vi "Create 3D Sphere.vi"(1 "Radius":sgl, 2 "Color":T1, 3 "Name":string) -> (0 "Scene:New Object":refnum<vi>)   [LabVIEW 2010]
uses:
  <vilib>/picture/3D Picture Control/NI_3D Picture Control.lvlib
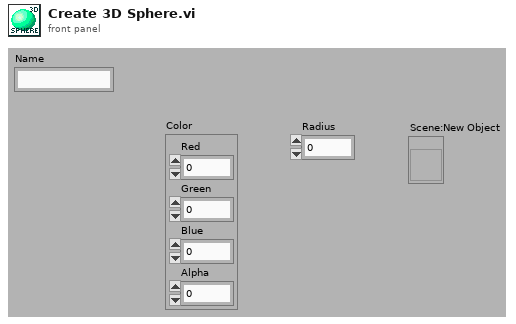
[diagram p1: front panel]
types:
  T1 = cluster{"Red":sgl, "Green":sgl, "Blue":sgl, "Alpha":sgl}
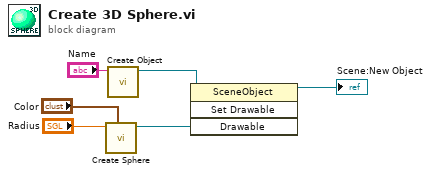
[diagram p0: block diagram]
diagram:
  n1 = call <vilib>:"Create Sphere.vi"("Color"="Color", "Radius"="Radius") -> ("New Sphere Refnum"=w4:refnum<vi>)  [unwired: 8 in, 1 out]
  n2 = call <vilib>:"Create Object.vi"("Name"="Name") -> ("Scene:New Object"=w2:refnum<vi>)  [unwired: 9 in, 1 out]
  n3 = invoke class="SceneObject" method="Set Drawable"(reference=w2, "Drawable"=w4) -> (reference out=→"Scene:New Object":refnum<vi>)  [unwired: 2 in, 3 out]
